vi "FGV_main.vi"(7 "FGV_mods":T2, 8 "Error In":errorcluster, 11 "DataIn":variant) -> (0 "Error Out":errorcluster, 2 "hits":T1[](array[typedef]), 3 "DataOut":variant)   [LabVIEW 2018]
uses:
  FGV_mods.ctl
  AE/hit_data.ctl
  FGV_data.ctl
  Config/config_data.ctl
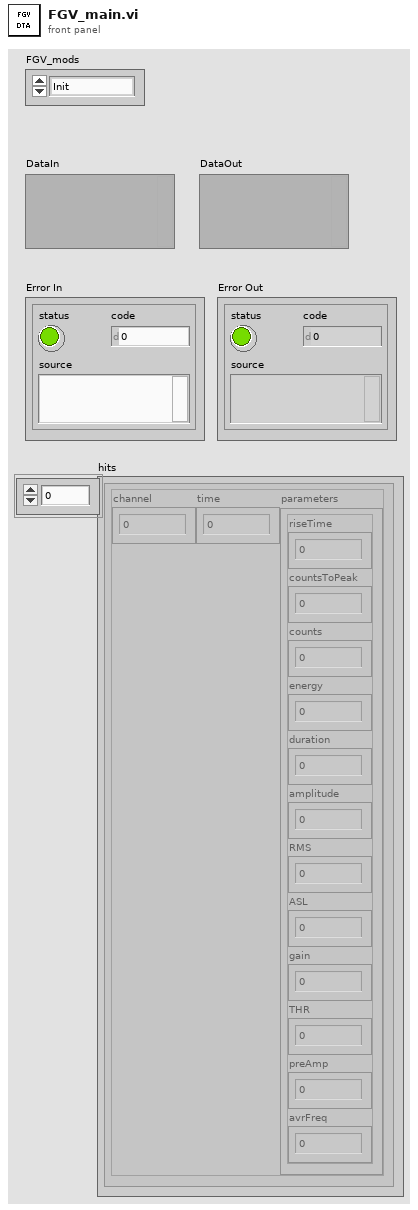
[diagram p1: front panel]
types:
  T1 = typedef "hit_data.ctl" = cluster{"channel":u8, "time":dbl, "parameters":cluster{"riseTime":u32, "countsToPeak":u32, "counts":u32, "energy":u32, "duration":u32, "amplitude":u32, "RMS":u32, "ASL":u32, "gain":u32, "THR":u32, "preAmp":u32, "avrFreq":u32}}
  T2 = typedef "FGV_mods.ctl" = enum16{"Init", "get_config", "get_hits", "set_file", "open_file", "close"}
  T3 = typedef "FGV_data.ctl" = cluster{"file":path, "time_coef":dbl, "config_data":T4, "file_ref":refnum<file>, "caller_VI":refnum<vi>}
  T4 = typedef "config_data.ctl" = cluster{"Size":i32[], "ID":u8[], "Parameter":string[], "testStart":timestamp, "testStart":u64}
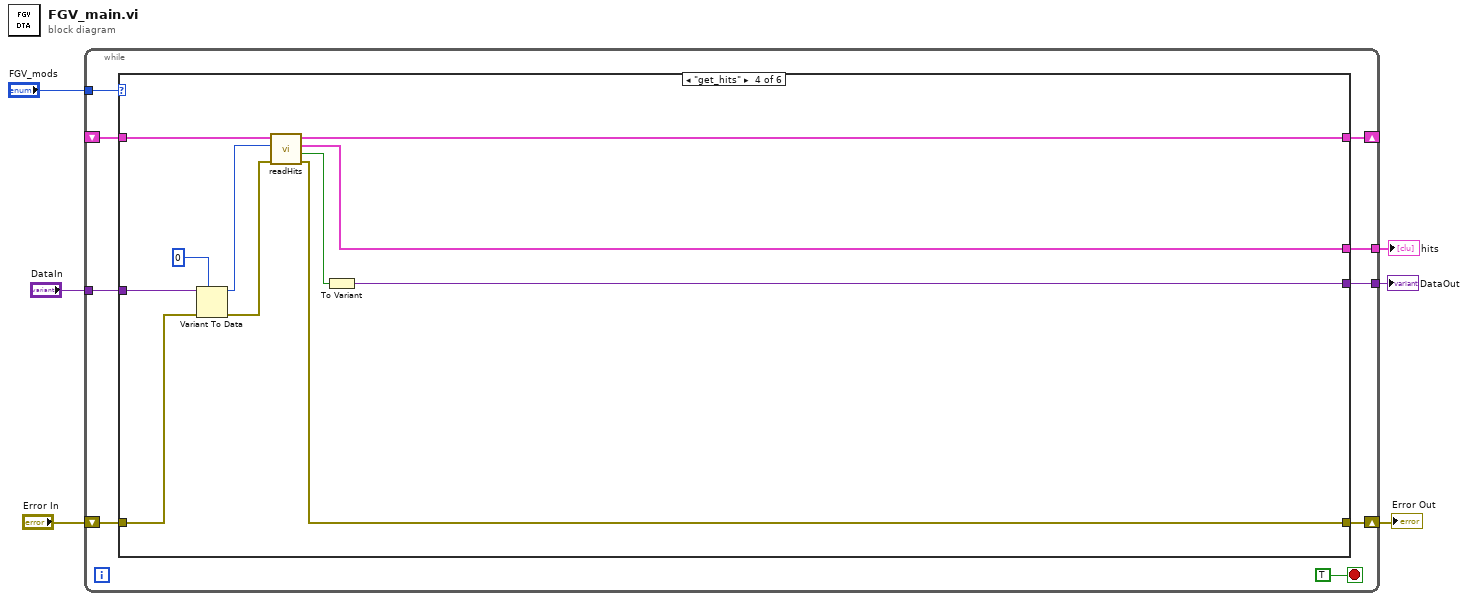
[diagram p0: block diagram]
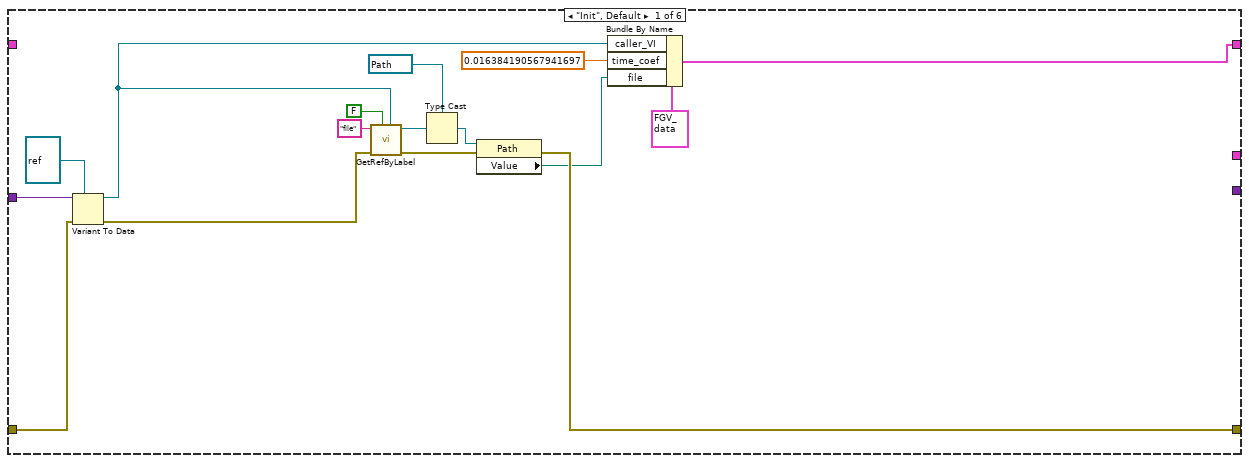
[diagram p2: hidden frame]
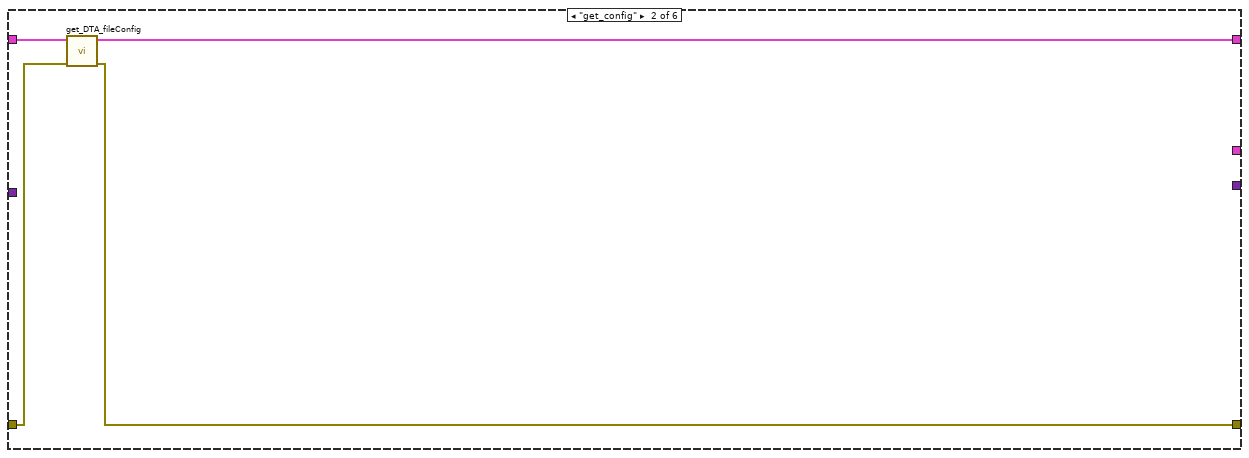
[diagram p3: hidden frame]
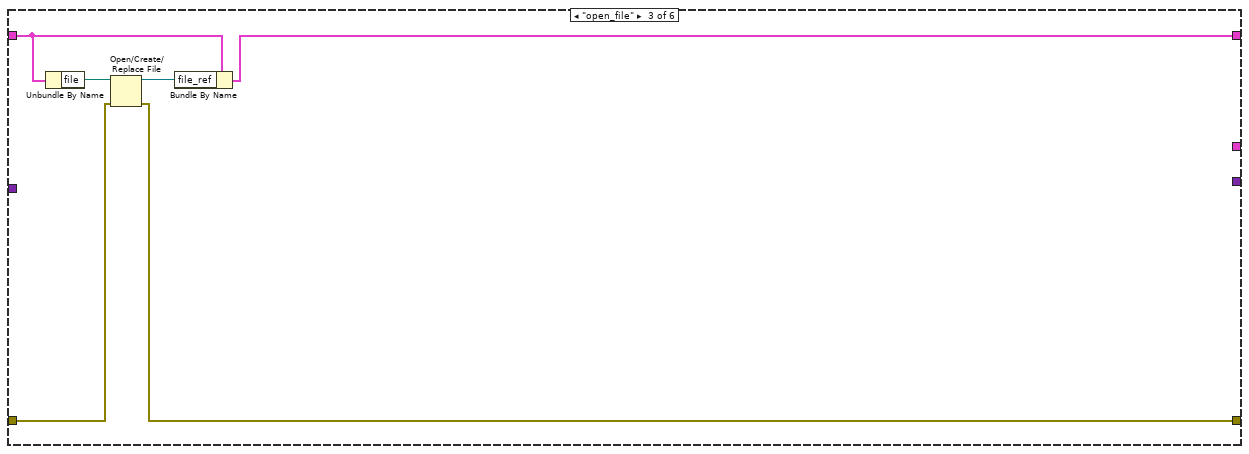
[diagram p4: hidden frame]
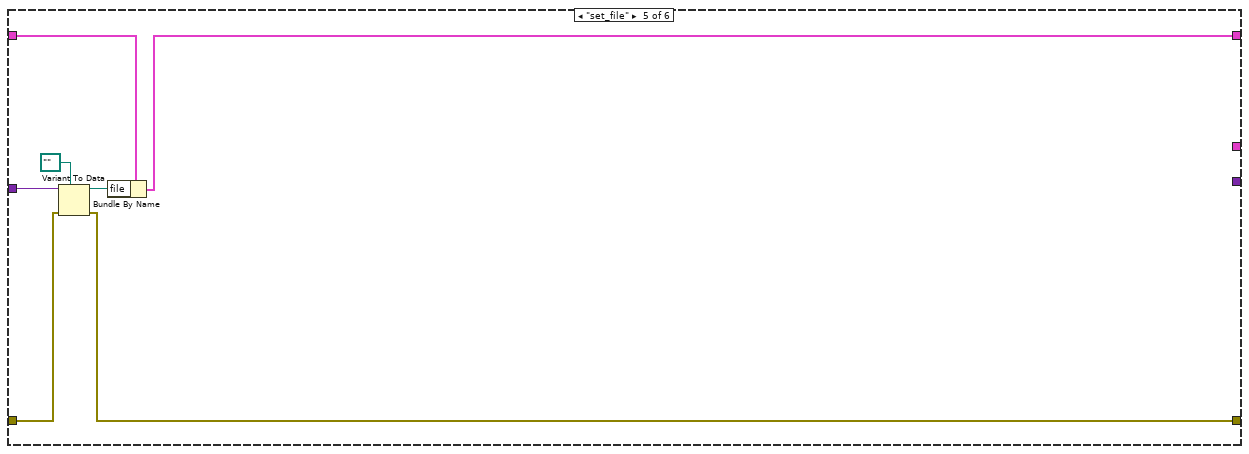
[diagram p5: hidden frame]
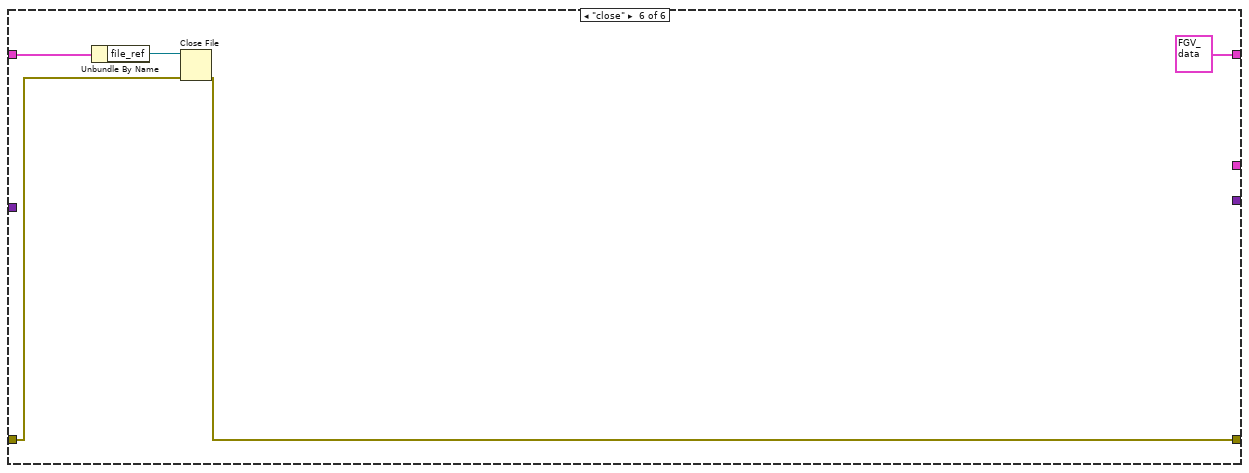
[diagram p6: hidden frame]
diagram:
  n1 = while {
    tunnel: "DataIn" -> [w14]
    tunnel: "FGV_mods" -> [w13]
    shift-right: [w12] -> _
    shift-left: _ -> [w11]
    shift-right: [w9] -> w3
    shift-left: "Error In" -> [w10]
    tunnel: [w8] -> w2
    tunnel: [w7] -> w1
    stop <- TRUE stop-if-true
    n2 = case shown="\"get_hits\"" w13 {
      tunnel: w14 -> [w22 _ _ w52 w59 _]
      tunnel: [w24 w33 w36 w46 w53 T3 {"file"=path "", "time_coef"=0.0, "config_data"={"Size"=[], "ID"=[], "Parameter"=[], "testStart"=timestamp(0 s since 1904-01-01), "testStart"=0}, "file_ref"=refnum, "caller_VI"=refnum} ("FGV_data out")] -> w12
      tunnel: w11 -> [_ w35 w38 w49 w55 w64]
      tunnel: w10 -> [w20 w34 w40 w50 w57 w62]
      tunnel: [w25 w32 w39 w47 w56 w61] -> w9
      tunnel: [_ _ _ w44 _ _] -> w8
      tunnel: [_ _ _ w43 _ _] -> w7
      frame "Init", Default {
        n3 = Variant To Data(error in=w20, type=refnum<vi> refnum ("This VI"), Variant=w22) -> (data=w18:refnum<vi>, error out=w19:errorcluster)
        n4 = call "GetRefByLabel.vi"("refVI"=w18, "InsideTab"=FALSE, "error in"=w19, "Label"="file") -> ("error out"=w26:errorcluster, "Ctl Refnum"=w30:refnum<vi>)  [unwired: 5 in, 1 out]
        n5 = Type Cast(type=refnum<vi> refnum ("file"), x=w30) -> (*(type *) &x=w27:refnum<vi>)
        n6 = property class="Path"(reference=w27, error in=w26) -> (error out=w25:errorcluster, "Value"=w17:path)  [unwired: 1 out]
        n7 = Bundle By Name(cluster=T3 {"file"=path "", "time_coef"=0.0, "config_data"={"Size"=[], "ID"=[], "Parameter"=[], "testStart"=timestamp(0 s since 1904-01-01), "testStart"=0}, "file_ref"=refnum, "caller_VI"=refnum} ("FGV_data"), "caller_VI"=w18, "time_coef"=0.016384190567941697 ("slope"), "file"=w17) -> (w24:T3)
      }
      frame "get_config" {
        n8 = call "get_DTA_fileConfig.vi"("Error In"=w34, "FGV_data"=w35) -> ("Error Out"=w32:errorcluster, "FGV_data out"=w33:T3)  [unwired: 8 in]
      }
      frame "open_file" {
        n9 = Unbundle By Name(w38) -> ("file"=w41:path)
        n10 = Open/Create/Replace File(file path (use dialog)=w41, error in=w40) -> (refnum out=w37:refnum<file>, error out=w39:errorcluster)  [unwired: 4 in, 1 out]
        n11 = Bundle By Name(cluster=w38, "file_ref"=w37) -> (w36:T3)
      }
      frame "get_hits" {
        n12 = Variant To Data(error in=w50, type=0, Variant=w52) -> (data=w42:i32, error out=w48:errorcluster)
        n13 = call "readHits.vi"("Error In"=w48, "#hits"=w42, "FGV_data"=w49) -> ("Error Out"=w47:errorcluster, "EOF"=w45:bool, "hits"=w43:T1[], "FGV_data out"=w46:T3)  [unwired: 5 in]
        n14 = To Variant(anything=w45) -> (Variant=w44:variant)
      }
      frame "set_file" {
        n15 = Variant To Data(error in=w57, type=path "", Variant=w59) -> (data=w54:path, error out=w56:errorcluster)
        n16 = Bundle By Name(cluster=w55, "file"=w54) -> (w53:T3)
      }
      frame "close" {
        n17 = Unbundle By Name(w64) -> ("file_ref"=w63:refnum<file>)
        n18 = Close File(refnum=w63, error in=w62) -> (error out=w61:errorcluster)  [unwired: 1 out]
      }
    }
  }
  "DataOut" <- w2
  "Error Out" <- w3
  "hits" <- w1
